vi "Write RFFE Waveform.vi"(5 "Reg_Address_Data":T1={"Address"=81, "Data"=0} {"Address" format="%.0x"}, 7 "USID":T2 max=15, 8 "error in (no error)":errorcluster, 11 "instrument handle":refnum<k15> caption="HSDIO_VISA") -> (0 "error out":errorcluster, 2 "Digital Waveform Graph":digitalwaveform(graph)={"t0"=timestamp(3585852840.1106524 s since 1904-01-01), "dt"=5e-07, "Y"={"transitions"=[], "data"=[[1, 0, 1, 0], [1, 0, 1, 0], [1, 0, 1, 0], [1, 0, 1, 0], [1, 0, 1, 0], [1, 0, 1, 0], [1, 0, 1, 0], [1, 0, 1, 0], [0, 0, 0, 0], [0, 0, 0, 0], [0, 0, 0, 0], [0, 0, 0, 0], [0, 0, 0, 0], [0, 0, 0, 0], [0, 0, 0, 0], [0, 0, 0, 0], [0, 1, 0, 1], [0, 1, 0, 1], [0, 1, 0, 1], [0, 1, 0, 1], [0, 0, 0, 0], [0, 0, 0, 0], [0, 0, 0, 0], [0, 0, 0, 0], [1, 1, 1, 1], [1, 1, 1, 1], [1, 1, 1, 1], [1, 1, 1, 1], [1, 0, 1, 0], [1, 0, 1, 0], [1, 0, 1, 0], [1, 0, 1, 0], [1, 1, 1, 1], [1, 1, 1, 1], [1, 1, 1, 1], [1, 1, 1, 1], [1, 0, 1, 0], [1, 0, 1, 0], [1, 0, 1, 0], [1, 0, 1, 0], [0, 1, 0, 1], [0, 1, 0, 1], [0, 1, 0, 1], [0, 1, 0, 1], [0, 0, 0, 0], [0, 0, 0, 0], [0, 0, 0, 0], [0, 0, 0, 0], [0, 1, 0, 1], [0, 1, 0, 1], [0, 1, 0, 1], [0, 1, 0, 1], [0, 0, 0, 0], [0, 0, 0, 0], [0, 0, 0, 0], [0, 0, 0, 0], [1, 1, 1, 1], [1, 1, 1, 1], [1, 1, 1, 1], [1, 1, 1, 1], [1, 0, 1, 0], [1, 0, 1, 0], [1, 0, 1, 0], [1, 0, 1, 0], [0, 1, 0, 1], [0, 1, 0, 1], [0, 1, 0, 1], [0, 1, 0, 1], [0, 0, 0, 0], [0, 0, 0, 0], [0, 0, 0, 0], [0, 0, 0, 0], [1, 1, 1, 1], [1, 1, 1, 1], [1, 1, 1, 1], [1, 1, 1, 1], [1, 0, 1, 0], [1, 0, 1, 0], [1, 0, 1, 0], [1, 0, 1, 0], [1, 1, 1, 1], [1, 1, 1, 1], [1, 1, 1, 1], [1, 1, 1, 1], [1, 0, 1, 0], [1, 0, 1, 0], [1, 0, 1, 0], [1, 0, 1, 0], [1, 1, 1, 1], [1, 1, 1, 1], [1, 1, 1, 1], [1, 1, 1, 1], [1, 0, 1, 0], [1, 0, 1, 0], [1, 0, 1, 0], [1, 0, 1, 0], [0, 1, 0, 1], [0, 1, 0, 1], [0, 1, 0, 1], [0, 1, 0, 1], [0, 0, 0, 0], [0, 0, 0, 0], [0, 0, 0, 0], [0, 0, 0, 0], [0, 1, 0, 1], [0, 1, 0, 1], [0, 1, 0, 1], [0, 1, 0, 1], [0, 0, 0, 0], [0, 0, 0, 0], [0, 0, 0, 0], [0, 0, 0, 0], [1, 1, 1, 1], [1, 1, 1, 1], [1, 1, 1, 1], [1, 1, 1, 1], [1, 0, 1, 0], [1, 0, 1, 0], [1, 0, 1, 0], [1, 0, 1, 0], [1, 1, 1, 1], [1, 1, 1, 1], [1, 1, 1, 1], [1, 1, 1, 1], [1, 0, 1, 0], [1, 0, 1, 0], [1, 0, 1, 0], [1, 0, 1, 0], [0, 1, 0, 1], [0, 1, 0, 1], [0, 1, 0, 1], [0, 1, 0, 1], [0, 0, 0, 0], [0, 0, 0, 0], [0, 0, 0, 0], [0, 0, 0, 0], [0, 1, 0, 1], [0, 1, 0, 1], [0, 1, 0, 1], [0, 1, 0, 1], [0, 0, 0, 0], [0, 0, 0, 0], [0, 0, 0, 0], [0, 0, 0, 0], [0, 1, 0, 1], [0, 1, 0, 1], [0, 1, 0, 1], [0, 1, 0, 1], [0, 0, 0, 0], [0, 0, 0, 0], [0, 0, 0, 0], [0, 0, 0, 0], [0, 1, 0, 1], [0, 1, 0, 1], [0, 1, 0, 1], [0, 1, 0, 1], [0, 0, 0, 0], [0, 0, 0, 0], [0, 0, 0, 0], [0, 0, 0, 0], [0, 1, 0, 1], [0, 1, 0, 1], [0, 1, 0, 1], [0, 1, 0, 1], [0, 0, 0, 0], [0, 0, 0, 0], [0, 0, 0, 0], [0, 0, 0, 0], [0, 1, 0, 1], [0, 1, 0, 1], [0, 1, 0, 1], [0, 1, 0, 1], [0, 0, 0, 0], [0, 0, 0, 0], [0, 0, 0, 0], [0, 0, 0, 0], [0, 1, 0, 1], [0, 1, 0, 1], [0, 1, 0, 1], [0, 1, 0, 1], [0, 0, 0, 0], [0, 0, 0, 0], [0, 0, 0, 0], [0, 0, 0, 0], [0, 1, 0, 1], [0, 1, 0, 1], [0, 1, 0, 1], [0, 1, 0, 1], [0, 0, 0, 0], [0, 0, 0, 0], [0, 0, 0, 0], [0, 0, 0, 0], [0, 1, 0, 1], [0, 1, 0, 1], [0, 1, 0, 1], [0, 1, 0, 1], [0, 0, 0, 0], [0, 0, 0, 0], [0, 0, 0, 0], [0, 0, 0, 0], [1, 0, 1, 0], [1, 0, 1, 0], [1, 0, 1, 0], [1, 0, 1, 0], [1, 0, 1, 0], [1, 0, 1, 0], [1, 0, 1, 0], [1, 0, 1, 0], [0, 0, 0, 0], [0, 0, 0, 0], [0, 0, 0, 0], [0, 0, 0, 0], [0, 0, 0, 0], [0, 0, 0, 0], [0, 0, 0, 0], [0, 0, 0, 0], [0, 1, 0, 1], [0, 1, 0, 1], [0, 1, 0, 1], [0, 1, 0, 1], [0, 0, 0, 0], [0, 0, 0, 0], [0, 0, 0, 0], [0, 0, 0, 0], [1, 1, 1, 1], [1, 1, 1, 1], [1, 1, 1, 1], [1, 1, 1, 1], [1, 0, 1, 0], [1, 0, 1, 0], [1, 0, 1, 0], [1, 0, 1, 0], [1, 1, 1, 1], [1, 1, 1, 1], [1, 1, 1, 1], [1, 1, 1, 1], [1, 0, 1, 0], [1, 0, 1, 0], [1, 0, 1, 0], [1, 0, 1, 0], [0, 1, 0, 1], [0, 1, 0, 1], [0, 1, 0, 1], [0, 1, 0, 1], [0, 0, 0, 0], [0, 0, 0, 0], [0, 0, 0, 0], [0, 0, 0, 0], [0, 1, 0, 1], [0, 1, 0, 1], [0, 1, 0, 1], [0, 1, 0, 1], [0, 0, 0, 0], [0, 0, 0, 0], [0, 0, 0, 0], [0, 0, 0, 0], [1, 1, 1, 1], [1, 1, 1, 1], [1, 1, 1, 1], [1, 1, 1, 1], [1, 0, 1, 0], [1, 0, 1, 0], [1, 0, 1, 0], [1, 0, 1, 0], [1, 1, 1, 1], [1, 1, 1, 1], [1, 1, 1, 1], [1, 1, 1, 1], [1, 0, 1, 0], [1, 0, 1, 0], [1, 0, 1, 0], [1, 0, 1, 0], [1, 1, 1, 1], [1, 1, 1, 1], [1, 1, 1, 1], [1, 1, 1, 1], [1, 0, 1, 0], [1, 0, 1, 0], [1, 0, 1, 0], [1, 0, 1, 0], [1, 1, 1, 1], [1, 1, 1, 1], [1, 1, 1, 1], [1, 1, 1, 1], [1, 0, 1, 0], [1, 0, 1, 0], [1, 0, 1, 0], [1, 0, 1, 0], [1, 1, 1, 1], [1, 1, 1, 1], [1, 1, 1, 1], [1, 1, 1, 1], [1, 0, 1, 0], [1, 0, 1, 0], [1, 0, 1, 0], [1, 0, 1, 0], [0, 1, 0, 1], [0, 1, 0, 1], [0, 1, 0, 1], [0, 1, 0, 1], [0, 0, 0, 0], [0, 0, 0, 0], [0, 0, 0, 0], [0, 0, 0, 0], [0, 1, 0, 1], [0, 1, 0, 1], [0, 1, 0, 1], [0, 1, 0, 1], [0, 0, 0, 0], [0, 0, 0, 0], [0, 0, 0, 0], [0, 0, 0, 0], [0, 1, 0, 1], [0, 1, 0, 1], [0, 1, 0, 1], [0, 1, 0, 1], [0, 0, 0, 0], [0, 0, 0, 0], [0, 0, 0, 0], [0, 0, 0, 0], [0, 1, 0, 1], [0, 1, 0, 1], [0, 1, 0, 1], [0, 1, 0, 1], [0, 0, 0, 0], [0, 0, 0, 0], [0, 0, 0, 0], [0, 0, 0, 0], [1, 1, 5, 1], [1, 1, 5, 1], [1, 1, 5, 1], [1, 1, 5, 1], [1, 0, 4, 0], [1, 0, 5, 0], [1, 0, 5, 0], [1, 0, 5, 0], [0, 1, 5, 1], [0, 1, 5, 1], [0, 1, 5, 1], [0, 1, 5, 1], [0, 0, 3, 0], [0, 0, 5, 0], [0, 0, 5, 0], [0, 0, 5, 0], [0, 1, 5, 1], [0, 1, 5, 1], [0, 1, 5, 1], [0, 1, 5, 1], [0, 0, 3, 0], [0, 0, 5, 0], [0, 0, 5, 0], [0, 0, 5, 0], [0, 1, 5, 1], [0, 1, 5, 1], [0, 1, 5, 1], [0, 1, 5, 1], [0, 0, 3, 0], [0, 0, 5, 0], [0, 0, 5, 0], [0, 0, 5, 0], [0, 1, 5, 1], [0, 1, 5, 1], [0, 1, 5, 1], [0, 1, 5, 1], [0, 0, 3, 0], [0, 0, 5, 0], [0, 0, 5, 0], [0, 0, 5, 0], [0, 1, 5, 1], [0, 1, 5, 1], [0, 1, 5, 1], [0, 1, 5, 1], [0, 0, 3, 0], [0, 0, 5, 0], [0, 0, 5, 0], [0, 0, 5, 0], [0, 1, 5, 1], [0, 1, 5, 1], [0, 1, 5, 1], [0, 1, 5, 1], [0, 0, 3, 0], [0, 0, 5, 0], [0, 0, 5, 0], [0, 0, 5, 0], [0, 1, 5, 1], [0, 1, 5, 1], [0, 1, 5, 1], [0, 1, 5, 1], [0, 0, 3, 0], [0, 0, 5, 0], [0, 0, 5, 0], [0, 0, 5, 0], [0, 1, 5, 1], [0, 1, 5, 1], [0, 1, 5, 1], [0, 1, 5, 1], [0, 0, 3, 0], [0, 0, 5, 0], [0, 0, 5, 0], [0, 0, 5, 0], [0, 1, 0, 1], [0, 1, 0, 1], [0, 1, 0, 1], [0, 1, 0, 1], [0, 0, 0, 0], [0, 0, 0, 0], [0, 0, 0, 0], [0, 0, 0, 0]]}}, 3 "Converted Data":cluster{"USID":u8, "Register":u8, "Data":u8} {"Register" max=31 format="%.0x"; "USID" max=15 format="%.0x"})   [LabVIEW 2013]
uses:
  Controls/USID.ctl
  Controls/Reg_Address_Data.ctl
  Instruments/HSDIO/MIPI_RFFE/Ctrls/Configuration.ctl
  Instruments/HSDIO/MIPI_RFFE/Ctrls/ClockDataChannels.ctl
  Instruments/HSDIO/MIPI_RFFE/Ctrls/RegReadWrite.ctl
  Instruments/HSDIO/MIPI_RFFE/Ctrls/ExtendedRegReadWrite.ctl
  <instrlib>/niHSDIO/niHSDIO.llb/niHSDIO Write Named Waveform (WDT).vi
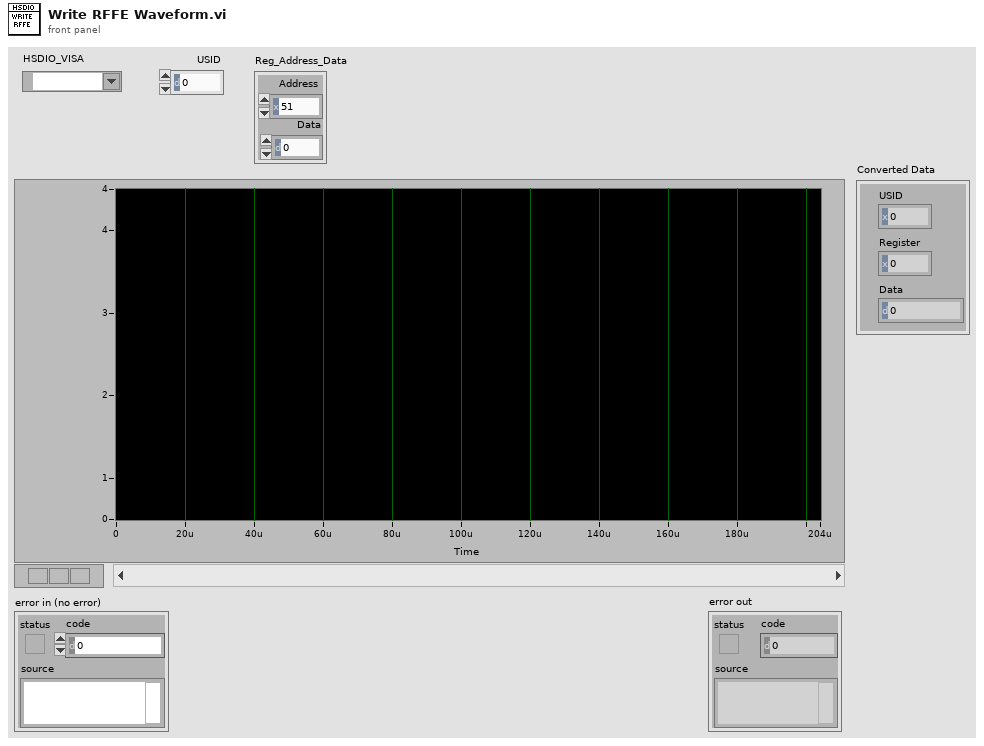
[diagram p1: front panel]
types:
  T1 = typedef "Reg_Address_Data.ctl" = cluster{"Address":u8, "Data":u8}
  T2 = typedef "USID.ctl" = u8
  T3 = typedef "RegReadWrite.ctl" = cluster{"Slave Address":u8, "Register":u8, "Data":u8, "SetID_Pin_State":enum16{"0", "1", "Z"}}
  T4 = typedef "Configuration.ctl" = cluster{"Samples to Allocate":i32, "Oversample Factor":u8, "Clock Channel":T5, "Data Channel":T5}
  T5 = typedef "ClockDataChannels.ctl" = enum16{"0", "1"}
  T6 = typedef "RFFE_Data.ctl" = cluster{"Clock Channel":T5, "Data Channel":T5, "Oversample Factor":u8, "Zero Array":u8[], "One Array":u8[], "Z Array ":u8[], "H Array":u8[], "L Array":u8[], "X Array":u8[], "Toggle (high to low)":u8[]}
  T7 = typedef "ExtendedRegReadWrite.ctl" = cluster{"Slave Address":u8, "Register":u8, "Data":u8[]}
  T8 = cluster{"Slave Address":u8, "Register":u8, "Data":u8}
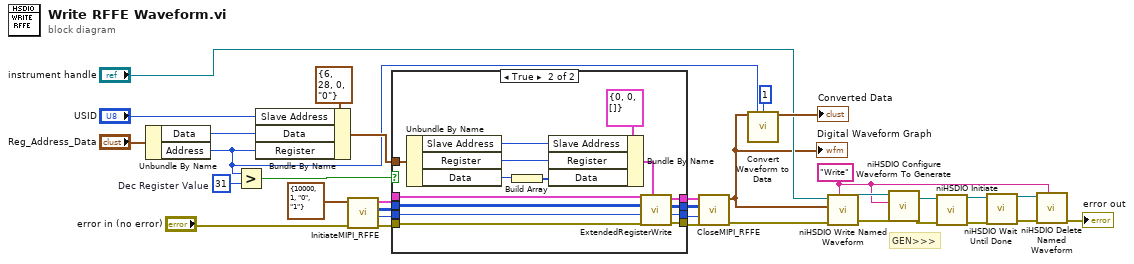
[diagram p0: block diagram]
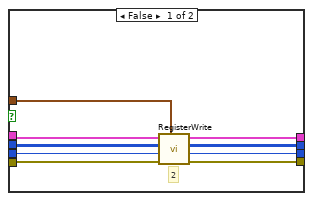
[diagram p2: hidden frame]
diagram:
  w5 = "Write" ("waveform name (default:\"\")")
  w32 = u8 31  # Dec Register Value
  # "GEN>>>"
  n1 = Unbundle By Name("Reg_Address_Data") -> ("Data"=w17:u8, "Address"=w16:u8)
  n2 = Greater?(x=w16, y=w32) -> (0:w26:bool)
  n3 = Bundle By Name(cluster=T3 {"Slave Address"=6, "Register"=28, "Data"=0, "SetID_Pin_State"=enum."0"} ("Data"), "Slave Address"="USID", "Data"=w17, "Register"=w16) -> (w20:T3)
  n4 = call "InitiateMIPI_RFFE.vi"("error in (no error)"="error in (no error)", "Configuratation In"=T4 {"Samples to Allocate"=10000, "Oversample Factor"=1, "Clock Channel"=enum."0", "Data Channel"=enum."1"} ("Configuratation")) -> ("error out"=w25:errorcluster, "Number of Samples Out"=w24:i32, "Data Array"=w23:u8[][], "RFFE_Data"=w22:T6)  [unwired: 6 in]
  n5 = case shown="True" w26 {
    tunnel: [w37 w47] -> w31
    tunnel: [w36 w48] -> w30
    tunnel: [w35 w49] -> w29
    tunnel: [w34 w50] -> w28
    tunnel: w20 -> [w42 w56]
    tunnel: w25 -> [w38 w46]
    tunnel: w24 -> [w39 w45]
    tunnel: w23 -> [w40 w44]
    tunnel: w22 -> [w41 w43]
    frame False {
      # "2"
      n6 = call "RegisterWrite.vi"("Write Data"=w42, "error in (no error)"=w38, "Number of Samples In"=w39, "Data Array"=w40, "RFFE_Data"=w41) -> ("error out"=w34:errorcluster, "Number of Samples Out"=w35:i32, "Data Array Out"=w36:u8[][], "Configuratation Out"=w37:T6)  [unwired: 3 in]
    }
    frame True {
      n7 = Unbundle By Name(w56) -> ("Slave Address"=w55:u8, "Register"=w54:u8, "Data"=w53:u8)
      n8 = Build Array(w53) -> (w52:u8[])
      n9 = Bundle By Name(cluster=T7 {"Slave Address"=0, "Register"=0, "Data"=[]} ("Extended Read/Write"), "Slave Address"=w55, "Register"=w54, "Data"=w52) -> (w51:T7)
      n10 = call "ExtendedRegisterWrite.vi"("Extended Read/Write"=w51, "error in (no error)"=w46, "Number of Samples In"=w45, "Data Array"=w44, "RFFE_Data In"=w43) -> ("error out"=w50:errorcluster, "Number of Samples Out"=w49:i32, "Data Array Out"=w48:u8[][], "RFFE_Data Out"=w47:T6)  [unwired: 3 in]
    }
  }
  n11 = call "CloseMIPI_RFFE.vi"("error in (no error)"=w28, "Number of Samples"=w29, "Data Array"=w30, "RFFE_Data"=w31) -> ("error out"=w3:errorcluster, "Digital Waveform"=w1:digitalwaveform)  [unwired: 6 in]
  "Digital Waveform Graph" <- w1
  n12 = call "Convert Waveform to Data.vi"("Waveform Graph"=w1, "Register"=w16, "Ext_Read_Num_Reg"=u8 1) -> ("Converted Data"=→"Converted Data":T8)  [unwired: 10 in, 2 out]
  n13 = call-poly <instrlib>:"niHSDIO Write Named Waveform.vi"("waveform name (default:\"\")"=w5, "error in (no error)"=w3, "data"=w1, "instrument handle"="instrument handle") -> ("error out"=w11:errorcluster, "instrument handle out"=w10:refnum<k15>)  [unwired: 6 in]
  n14 = call <instrlib>:"niHSDIO Configure Waveform To Generate.vi"("error in (no error)"=w11, "waveform name"=w5, "instrument handle"=w10) -> ("error out"=w8:errorcluster, "instrument handle out"=w9:refnum<k15>)  [unwired: 7 in]
  n15 = call <instrlib>:"niHSDIO Initiate.vi"("error in (no error)"=w8, "instrument handle"=w9) -> ("error out"=w13:errorcluster, "instrument handle out"=w12:refnum<k15>)  [unwired: 8 in]
  n16 = call <instrlib>:"niHSDIO Wait Until Done.vi"("error in (no error)"=w13, "instrument handle"=w12) -> ("error out"=w7:errorcluster, "instrument handle out"=w6:refnum<k15>)  [unwired: 8 in]
  n17 = call <instrlib>:"niHSDIO Delete Named Waveform.vi"("waveform name (default:\"\")"=w5, "error in (no error)"=w7, "instrument handle"=w6) -> ("error out"=→"error out":errorcluster)  [unwired: 7 in, 1 out]
